vi "Update CMDS.vi"(8 "error in (no error)":errorcluster, 10 "New Value":bool, 11 "Tag":T1) -> (0 "error out":errorcluster)   [LabVIEW 2018]
uses:
  CTL/Tags.ctl
  CTL/FGV - R-W.ctl
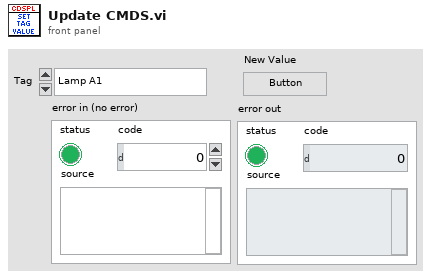
[diagram p1: front panel]
types:
  T1 = typedef "Tags.ctl" = enum16{"Lamp A1", "Lamp B1", "Lamp C1", "Lamp D1", "Lamp E1", "Lamp F1", "Lamp G1", "Lamp H1", "Lamp A2", "Lamp B2", "Lamp C2", "Lamp D2", "Lamp E2", "Lamp F2", "Lamp G2", "Lamp H2", "Ack A1", "Ack B1", "Ack C1", "Ack D1", "Ack E1", "Ack F1", "Ack G1", "Ack H1", "Ack A2", "Ack B2", "Ack C2", "Ack D2", "Ack E2", "Ack F2", "Ack G2", "Ack H2", "SSM", "SAS", "LSM", ""}
  T2 = typedef "FGV - R-W.ctl" = enum16{"W", "R"}
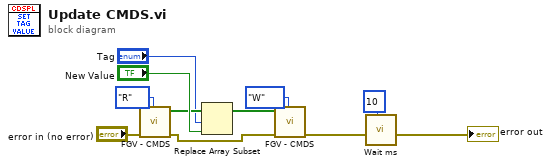
[diagram p0: block diagram]
diagram:
  n1 = call "FGV - CMDS.vi"("Action"=FGV_-_R-W."R", "error in (no error)"="error in (no error)") -> ("error out"=w6:errorcluster, "Cmd Out"=w9:bool[])  [unwired: 8 in]
  n2 = Replace Array Subset(array=w9, new element="New Value", index="Tag") -> (w7:bool[])
  n3 = call "FGV - CMDS.vi"("Action"=FGV_-_R-W."W", "error in (no error)"=w6, "Cmd In"=w7) -> ("error out"=w3:errorcluster)  [unwired: 7 in, 1 out]
  n4 = call "Wait ms.vi"("milliseconds to wait"=u32 10, "error in (no error)"=w3) -> ("error out"=→"error out":errorcluster)  [unwired: 9 in]
